vi "Get DispSnsr Value.vi"(8 "error in (no error)":errorcluster, 11 "VacuumLine in":refnum<class "VacuumLine.lvclass">) -> (0 "error out":errorcluster, 2 "distance":dbl, 3 "VacuumLine out":refnum<class "VacuumLine.lvclass">)   [LabVIEW 2016, in "Hardware.lvlib" / "VacuumLine.lvlib" / "VacuumLine.lvclass"]
uses:
  <userlib>/Common Components/Hardware/Abstract System/VacuumLine/VacuumLine/VacuumLine.lvclass
  <userlib>/Common Components/Hardware/Abstract System/VacuumLine/VacuumLine/VacuumLine.lvclass/VacuumLine.ctl
  <userlib>/Common Components/Hardware/Displacement Sensor/DispSnsr/DispSnsr.lvclass
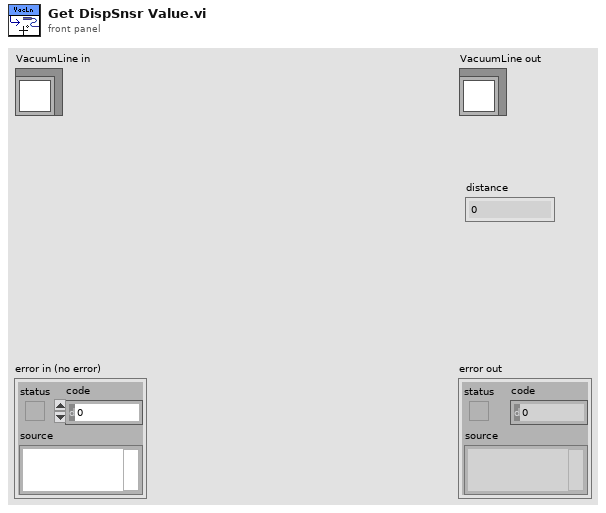
[diagram p1: front panel]
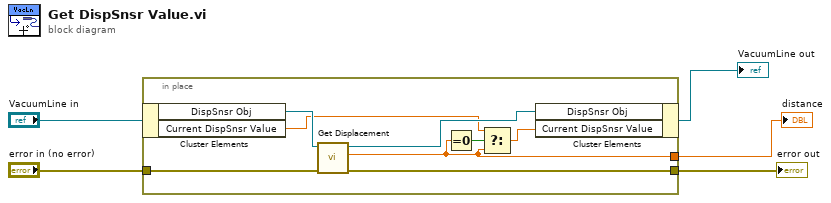
[diagram p0: block diagram]
diagram:
  n1 = in-place {
    in-place-border: "error in (no error)" -> [w13]
    in-place-border: [w12] -> w4
    in-place-border: [w7] -> w3
    n2 = in-place-cluster #1("VacuumLine in") -> ("DispSnsr Obj"=w11:refnum<class "DispSnsr.lvclass">, "Current DispSnsr Value"=w8:dbl)
    n3 = call-dynamic "Get Displacement.vi"("error in (no error)"=w13, "Displacement Sensor in"=w11) -> ("error out"=w12:errorcluster, "Displacement"=w7:dbl, "Displacement Sensor out"=w10:refnum<class "DispSnsr.lvclass">)  [unwired: 7 in]
    n4 = Equal To 0?(x=w7) -> (x = 0?=w9:bool)
    n5 = Select(t=w8, s=w9, f=w7) -> (s? t:f=w6:dbl)
    n6 = in-place-cluster #1("DispSnsr Obj"=w10, "Current DispSnsr Value"=w6) -> (→"VacuumLine out":refnum<class "VacuumLine.lvclass">)
  }
  "error out" <- w4
  "distance" <- w3
